vi "Clear Tree.vi"(8 "error in (no error)":errorcluster, 11 "Tag Tree Helper In":refnum<class "Tag Tree Helper.lvclass">) -> (0 "error out":errorcluster, 3 "Tag Tree Helper Out":refnum<class "Tag Tree Helper.lvclass">)   [LabVIEW 2020, in "Process Generation.lvlib" / "Tag Tree Helper.lvclass"]
uses:
  Tag Tree Helper.lvclass
  Tag Tree Helper.lvclass/Tag Tree Helper.ctl
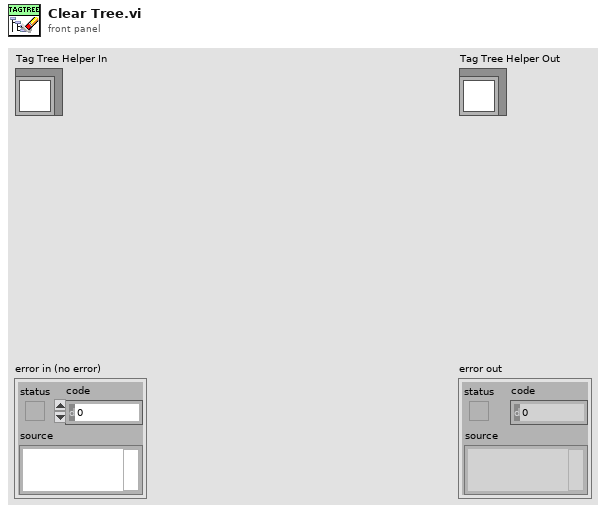
[diagram p1: front panel]
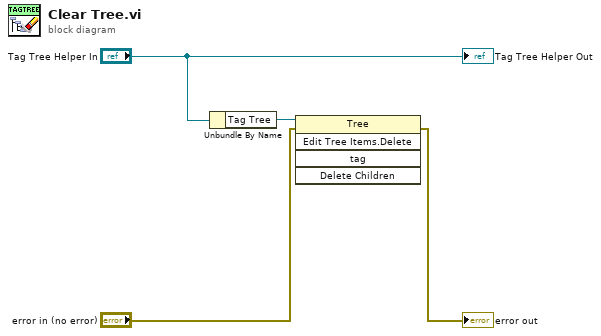
[diagram p0: block diagram]
diagram:
  n1 = Unbundle By Name("Tag Tree Helper In") -> ("Tag Tree"=w3:refnum<vi>)
  n2 = invoke class="Tree" method="Edit Tree Items.Delete"(reference=w3, error in="error in (no error)") -> (error out=→"error out":errorcluster)  [unwired: 3 in, 4 out]
  "Tag Tree Helper Out" <- "Tag Tree Helper In"
